vi "Clicked.vi"(0 "reference in":refnum<class "Pgui_Obj.lvclass">, 5 "error in (no error)":errorcluster) -> (14 "reference out":refnum<class "Pgui_Obj.lvclass">, 15 "Array":string[](array[string]), 19 "error out":errorcluster)   [LabVIEW 2019, in "Pgui_Obj.lvclass"]
uses:
  Pgui_Obj.lvclass
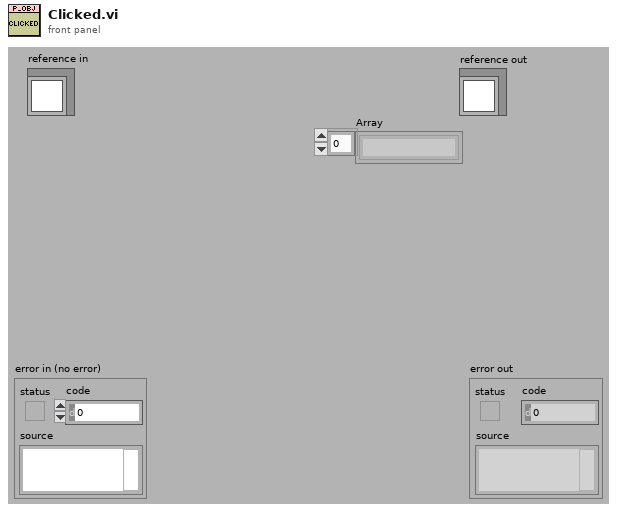
[diagram p1: front panel]
types:
  T1 = typedef "Pgui_Obj.lvclass/ObjectAttributes.ctl" = cluster{"Children":refnum<class "Pgui_Obj.lvclass">[], "Draw Instr":picture, "Params":cluster{"left":i16, "top":i16, "right":i16, "bottom":i16}, "Parent_Pgui_Obj":refnum<class "Pgui_Obj.lvclass">, "MouseOver":bool}
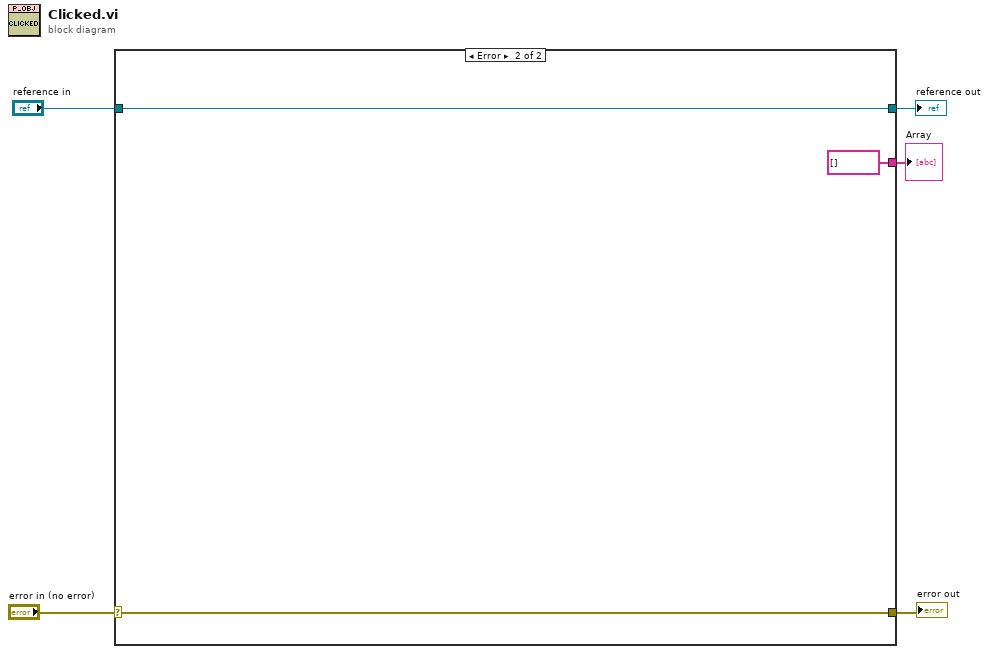
[diagram p0: block diagram]
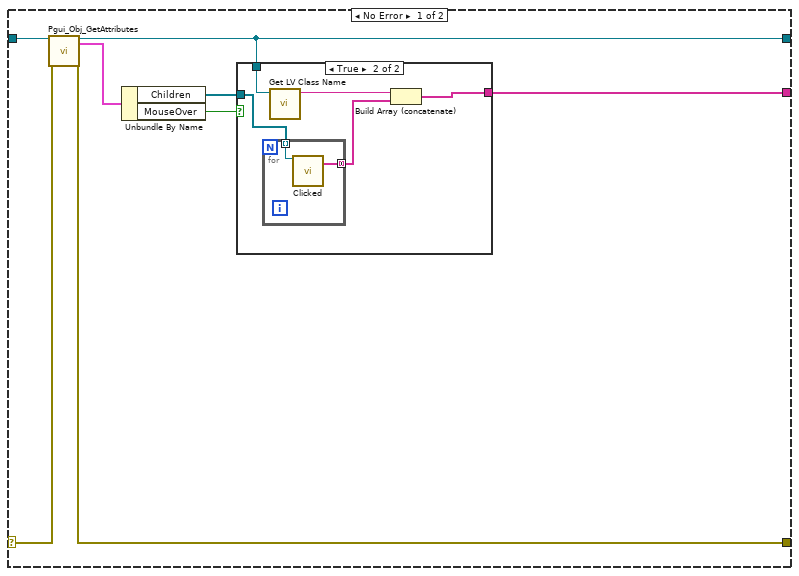
[diagram p2: hidden frame]
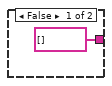
[diagram p3: hidden frame]
diagram:
  n1 = case shown="Error" "error in (no error)" {
    selector: "error in (no error)" -> [w13 w24]
    tunnel: [w11 w24] -> w4
    tunnel: [w8 w23] -> w2
    tunnel: "reference in" -> [w10 w23]
    tunnel: [w7 string[] []] -> w1
    frame No Error {
      n2 = call "Pgui_Obj_GetAttributes.vi"("reference in"=w10, "error in (no error)"=w13) -> ("reference out"=w8:refnum<class "Pgui_Obj.lvclass">, "Data"=w12:T1, "error out"=w11:errorcluster)  [unwired: 14 in, 1 out]
      n3 = Unbundle By Name(w12) -> ("Children"=w6:refnum<class "Pgui_Obj.lvclass">[], "MouseOver"=w9:bool)
      n4 = case shown="True" w9 {
        tunnel: w8 -> [_ w19]
        tunnel: [string[] [] w17] -> w7
        tunnel: w6 -> [_ w16]
        frame False {
        }
        frame True {
          n5 = for {
            tunnel: w16 -> [w21] mode=indexing
            tunnel: [w20] -> w15 mode=concatenating
            n6 = call-dynamic "Clicked.vi"("reference in"=w21) -> ("Array"=w20:string[])  [unwired: 16 in, 2 out]
          }
          n7 = call <vilib>:"Get LV Class Name.vi"("object"=w19) -> ("class name"=w18:string)  [unwired: 9 in, 1 out]
          n8 = Build Array (concatenate)(w18, w15) -> (w17:string[])
        }
      }
    }
    frame Error {
    }
  }
  "error out" <- w4
  "reference out" <- w2
  "Array" <- w1
